vi "Add Library To Project.vi"(8 "error in":errorcluster, 11 "Actor Script Strategy in":refnum<class "Actor Script Strategy.lvclass">) -> (0 "error out":errorcluster)   [LabVIEW 2021, in "_Create From Template.lvlib" / "Script Strategy.lvlib" / "Actor Script Strategy.lvclass"]
uses:
  Actor Script Strategy.lvclass
  Actor Script Strategy.lvclass/Actor Script Strategy.ctl
  <vilib>/Utility/EditLVLibs/Edit LVLibs.lvlib
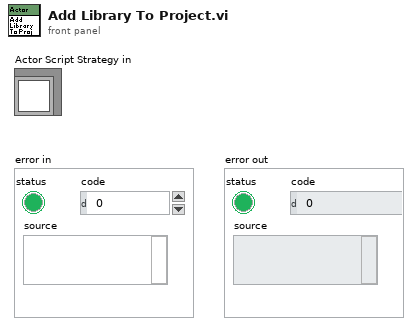
[diagram p1: front panel]
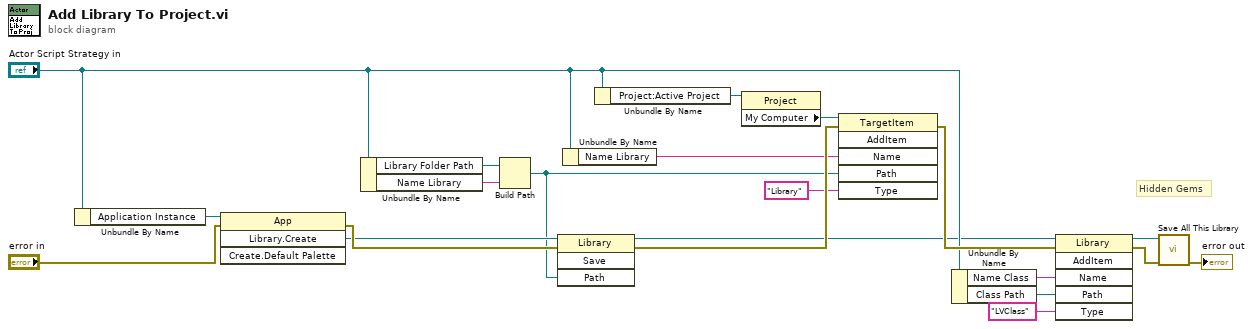
[diagram p0: block diagram]
diagram:
  # "Hidden Gems"
  n1 = Unbundle By Name("Actor Script Strategy in") -> ("Application Instance"=w12:refnum<vi>)
  n2 = invoke class="App" method="Library.Create"(reference=w12, error in="error in") -> (error out=w17:errorcluster, "Create Library"=w14:refnum<vi>)  [unwired: 2 in, 2 out]
  n3 = Unbundle By Name("Actor Script Strategy in") -> ("Library Folder Path"=w10:path, "Name Library"=w5:string)
  n4 = Build Path(base path=w10, name or relative path=w5) -> (appended path=w1:path)
  n5 = invoke class="Library" method="Save"(reference=w14, error in=w17, "Path"=w1) -> (reference out=w2:refnum<vi>, error out=w16:errorcluster)  [unwired: 1 in, 2 out]
  n6 = Unbundle By Name("Actor Script Strategy in") -> ("Name Library"=w3:string)
  n7 = Unbundle By Name("Actor Script Strategy in") -> ("Project:Active Project"=w11:refnum<vi>)
  n8 = property class="Project"(reference=w11) -> ("My Computer"=w13:refnum<vi>)  [unwired: 1 in, 2 out]
  n9 = invoke class="TargetItem" method="AddItem"(reference=w13, error in=w16, "Name"=w3, "Path"=w1, "Type"="Library") -> (error out=w19:errorcluster)  [unwired: 1 in, 5 out]
  n10 = Unbundle By Name("Actor Script Strategy in") -> ("Name Class"=w7:string, "Class Path"=w6:path)
  n11 = invoke class="Library" method="AddItem"(reference=w2, error in=w19, "Name"=w7, "Path"=w6, "Type"="LVClass") -> (reference out=w8:refnum<vi>, error out=w20:errorcluster)  [unwired: 1 in, 4 out]
  n12 = call <vilib>:"Save All This Library.vi"("error in (no error)"=w20, "Library in"=w8) -> ("error out"=→"error out":errorcluster)  [unwired: 8 in, 1 out]
